vi "Init Events.vi"(8 "error in (no error)":errorcluster, 11 "RemoteDataService in":refnum<class "RemoteDataService.lvclass">) -> (0 "error out":errorcluster, 3 "RemoteDataService out":refnum<class "RemoteDataService.lvclass">)   [LabVIEW 2020, in "Vecto.lvlib" / "RemoteDataService.lvclass"]
uses:
  RemoteDataService.lvclass
  Register Group Data.ctl
  Group/Group.lvclass
  Incoming Events.ctl
  Publish Group Data.ctl
  proto/GroupData/Class/Msg.lvclass
  Subscribe Data.ctl
  Subscription.ctl
  Registered Groups Data.ctl
  lv-promises/Promises/Promise/Promise.lvclass
  RemoteDataService.lvclass/RemoteDataService.ctl
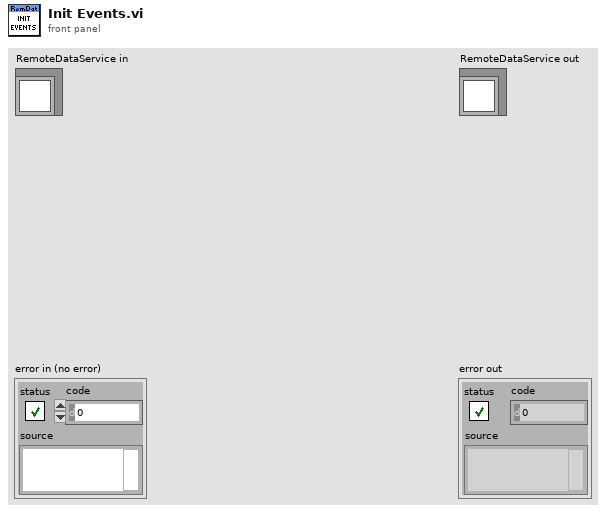
[diagram p1: front panel]
types:
  T1 = typedef "Vecto.lvlib/RemoteDataService.lvclass/Registered Groups Data.ctl" = cluster{"Promise":refnum<class "Promise.lvclass">}
  T2 = typedef "Vecto.lvlib/RemoteDataService.lvclass/Subscribe Data.ctl" = cluster{"Subscription":T3}
  T3 = typedef "Vecto.lvlib/RemoteDataService.lvclass/Subscription.ctl" = cluster{"Multicast Address":string, "Multicast Port":u16}
  T4 = typedef "Vecto.lvlib/RemoteDataService.lvclass/Publish Group Data.ctl" = cluster{"GroupData":refnum<class "Msg.lvclass">}
  T5 = typedef "Vecto.lvlib/RemoteDataService.lvclass/Incoming Events.ctl" = cluster{"Register Group":refnum<user-event>, "Close":refnum<user-event>, "Publish Group":refnum<user-event>, "Start":refnum<user-event>, "Subscribe":refnum<user-event>, "Registered Groups":refnum<user-event>}
  T6 = typedef "Vecto.lvlib/RemoteDataService.lvclass/Register Group Data.ctl" = cluster{"Group":refnum<class "Group.lvclass">}
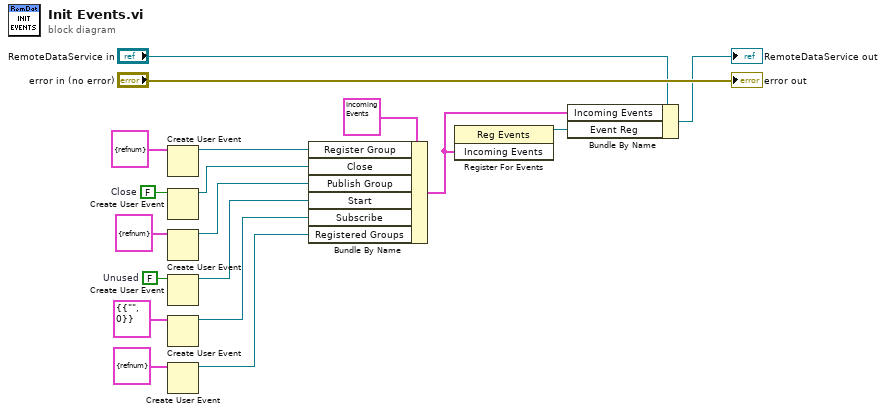
[diagram p0: block diagram]
diagram:
  w6 = FALSE  # Unused
  w10 = FALSE  # Close
  n1 = Create User Event(user event datatype=T6 {"Group"=refnum} ("Register Group Data")) -> (user event=w15:refnum<user-event>)  [unwired: 1 in, 1 out]
  n2 = Create User Event(user event datatype=w10) -> (user event=w9:refnum<user-event>)  [unwired: 1 in, 1 out]
  n3 = Create User Event(user event datatype=T4 {"GroupData"=refnum} ("Publish Group Data")) -> (user event=w7:refnum<user-event>)  [unwired: 1 in, 1 out]
  n4 = Create User Event(user event datatype=w6) -> (user event=w5:refnum<user-event>)  [unwired: 1 in, 1 out]
  n5 = Create User Event(user event datatype=T2 {"Subscription"={"Multicast Address"="", "Multicast Port"=0}} ("Subscribe Data")) -> (user event=w3:refnum<user-event>)  [unwired: 1 in, 1 out]
  n6 = Create User Event(user event datatype=T1 {"Promise"=refnum} ("Registered Groups Data")) -> (user event=w1:refnum<user-event>)  [unwired: 1 in, 1 out]
  n7 = Bundle By Name(cluster=T5 {"Register Group"=refnum, "Close"=refnum, "Publish Group"=refnum, "Start"=refnum, "Subscribe"=refnum, "Registered Groups"=refnum} ("Incoming Events"), "Register Group"=w15, "Close"=w9, "Publish Group"=w7, "Start"=w5, "Subscribe"=w3, "Registered Groups"=w1) -> (w13:T5)
  n8 = register-events(w13) -> (reference out=w14:refnum<event-registration>)  [unwired: 2 in, 1 out]
  n9 = Bundle By Name(cluster="RemoteDataService in", "Incoming Events"=w13, "Event Reg"=w14) -> (→"RemoteDataService out":refnum<class "RemoteDataService.lvclass">)
  "error out" <- "error in (no error)"
